vi "Subspaces Angle (2D 1D).vi"(10 "B":dbl[](array[numeric]), 11 "A":T1) -> (0 "error":i32, 3 "angle":dbl)   [LabVIEW 2017, in "NI_AAL_LinAlg.lvlib"]
doc: "Computes the angle between column spaces of two matrices."
uses:
  <vilib>/Analysis/NI_AAL_LinAlg.lvlib
  <vilib>/Analysis/Matrix/Datatypes/RealMatrix.ctl
  <vilib>/Analysis/7linalg.llb/SVD Option.ctl
  <vilib>/Analysis/baseanly.llb/Unit Vector (DBL).vi
  <vilib>/Analysis/7linalg.llb/Real Transpose Matrix.vi
  <vilib>/Analysis/baseanly.llb/A x Vector.vi
  <vilib>/Analysis/7linalg.llb/Real SVD Decomposition.vi
  <vilib>/Analysis/NI_AALBase.lvlib
  <vilib>/Analysis/NI_AALPro.lvlib
  <vilib>/Analysis/Matrix/NI_Matrix.lvlib
panel:
  # "Angle Between Subspaces (2D, 1D)"
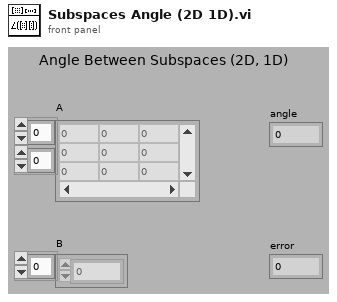
[diagram p1: front panel]
types:
  T1 = typedef "NI_Matrix.lvlib/RealMatrix.ctl" = dbl[][]
  T2 = typedef "NI_AALPro.lvlib/SVD Option.ctl" = u16
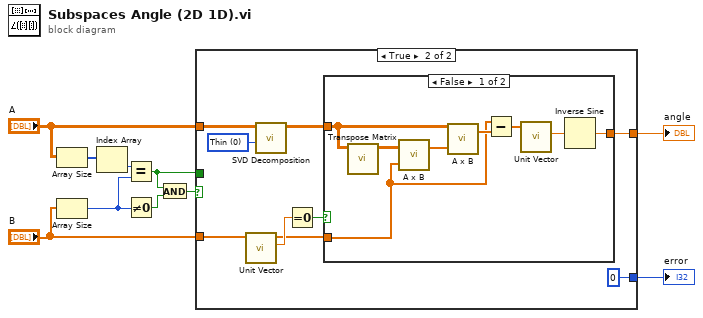
[diagram p0: block diagram]
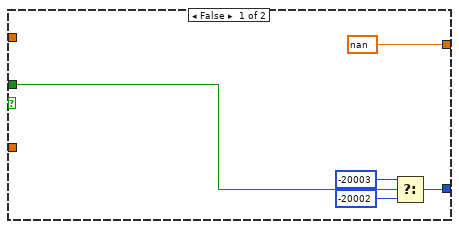
[diagram p2: hidden frame]
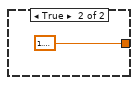
[diagram p3: hidden frame]
diagram:
  n1 = Array Size(array="A") -> (size(s)=w10:i32[])
  n2 = Array Size(array="B") -> (size(s)=w4:i32)
  n3 = Index Array(array=w10) -> (element=w9:i32)  [unwired: 1 in]
  n4 = Equal?(x=w9, y=w4) -> (x = y?=w1:bool)
  n5 = Not Equal To 0?(x=w4) -> (x != 0?=w3:bool)
  n6 = And(x=w1, y=w3) -> (x .and. y?=w2:bool)
  n7 = case shown="True" w2 {
    tunnel: "A" -> [_ w24]
    tunnel: "B" -> [_ w23]
    tunnel: [nan ("norm") w18] -> w7
    tunnel: [w14 0] -> w6
    tunnel: w1 -> [w11 _]
    frame False {
      n8 = Select(t=-20003, s=w11, f=-20002) -> (s? t:f=w14:i32)
    }
    frame True {
      w16 = T2 0 items=["Thin", "Full"] ("SVD option")
      n9 = call-poly <vilib>:"Unit Vector.vi"("Input Vector"=w23) -> ("norm"=w22:dbl, "Unit Vector"=w20:dbl[])  [unwired: 2 in, 7 out]
      n10 = call-poly <vilib>:"SVD Decomposition.vi"("SVD option"=w16, "A"=w24) -> ("Matrix U"=w19:T1)  [unwired: 1 in, 8 out]
      n11 = Equal To 0?(x=w22) -> (x = 0?=w21:bool)
      n12 = case shown="False" w21 {
        tunnel: w20 -> [w28 _]
        tunnel: w19 -> [w31 _]
        tunnel: [w25 1.5707963267948966 ("norm")] -> w18
        frame False {
          n13 = call-poly <vilib>:"Transpose Matrix.vi"("Input Matrix"=w31) -> ("Matrix Transpose"=w32:T1)  [unwired: 10 out]
          n14 = call-poly <vilib>:"A x B.vi"("Vector"=w28, "A"=w32) -> ("A x Vector"=w30:dbl[])  [unwired: 1 out]
          n15 = call-poly <vilib>:"A x B.vi"("Vector"=w30, "A"=w31) -> ("A x Vector"=w29:dbl[])  [unwired: 1 out]
          n16 = Subtract(x=w28, y=w29) -> (x-y=w27:dbl[])
          n17 = call-poly <vilib>:"Unit Vector.vi"("Input Vector"=w27) -> ("norm"=w26:dbl)  [unwired: 2 in, 8 out]
          n18 = Inverse Sine(1:w26) -> (0:w25:dbl)
        }
        frame True {
        }
      }
    }
  }
  "error" <- w6
  "angle" <- w7
